vi "Init Tree.vi"(11 "Tree In":refnum<vi>) -> (3 "Tree Out":refnum<vi>)   [LabVIEW 2019, in "Tree Browser.lvlib"]
doc: "Setup a tree for browsing directories on disk. Inserts a top level root node, then child nodes for each available disk (C:\\, D:\\, etc)."
uses:
  Tree Browser.lvlib
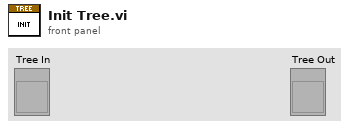
[diagram p1: front panel]
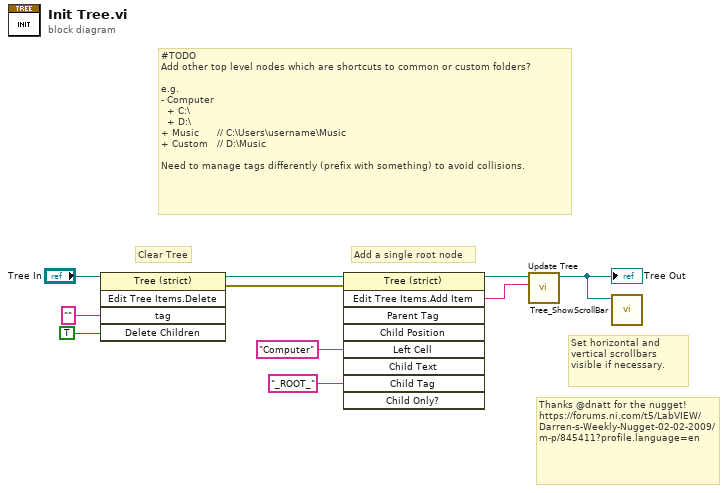
[diagram p0: block diagram]
diagram:
  # "#TODO\nAdd other top level nodes which are shortcuts to common or custom folders?\n\ne.g.\n- Computer\n  + C:\\\n  + D:\\\n+ Music      // C:\\Users\\username\\Music\n+ Custom   // D:\\Music\n\nNeed to manage tags differently (prefix with something) to avoid collisions."
  # "Thanks @dnatt for the nugget!\nhttps://forums.ni.com/t5/LabVIEW/Darren-s-Weekly-Nugget-02-02-2009/m-p/845411?profile.language=en"
  # "Set horizontal and vertical scrollbars visible if necessary."
  # "Add a single root node"
  # "Clear Tree"
  n1 = invoke class="Tree (strict)" method="Edit Tree Items.Delete"(reference="Tree In", "tag"="" ("Tag"), "Delete Children"=TRUE ("Delete Children?")) -> (reference out=w10:refnum<vi>, error out=w4:errorcluster)  [unwired: 2 in, 3 out]
  n2 = invoke class="Tree (strict)" method="Edit Tree Items.Add Item"(reference=w10, error in=w4, "Left Cell"="Computer" ("Left Cell String"), "Child Tag"="_ROOT_") -> (reference out=w2:refnum<vi>, "Edit Tree Items:Add Item"=w3:string)  [unwired: 5 in, 7 out]
  n3 = call "Update Tree.vi"("Parent Tag"=w3, "Tree In"=w2) -> ("Tree Out"=w1:refnum<vi>)  [unwired: 9 in]
  "Tree Out" <- w1
  n4 = call <vilib>:"Tree_ShowScrollBar.vi"("Tree"=w1) -> ()  [unwired: 10 in, 1 out]
